vi "Click Cycle_Update Value.vi"(7 "Action":T1, 8 "Error In":errorcluster, 9 "Save Action":T2(ring)=enum."Remove", 10 "Tag":string, 11 "Row RW State":T3) -> (0 "Error Out":errorcluster)   [LabVIEW 2023]
uses:
  controls/action enum.ctl
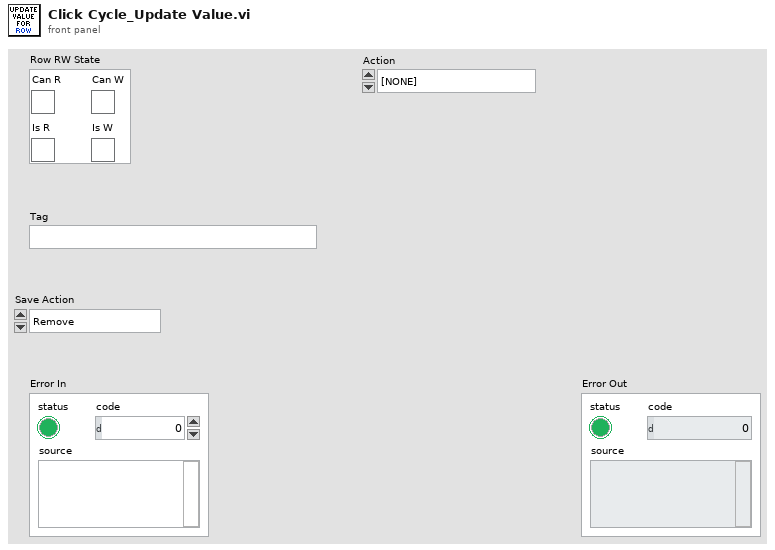
[diagram p1: front panel]
types:
  T1 = typedef "action enum.ctl" = enum16{"[NONE]", "Wire Bundle", "Wire Unbundle", "Terminal Unbundle", "Terminal Bundle", "Bundler Move Up", "Bundler Move Down", "Bundler Insert", "Bundler Remove", "Bundler Remove Unwired", "Bundler Rearrange", "In Place Insert", "In Place Remove", "In Place Remove Unwired", "In Place Rearrange", "Wire Properties", "Wire Method", "Terminal Properties", "Terminal Method", "Property Move Up", "Property Move Down", "Properties Insert", "Properties Remove", "Properties Remove Unwired", "Properties Rearrange", "Method Change", "Class for Constant", "Class For Control", "Class For Node", "Class Name to Clipboard"}
  T2 = enum16{"Init", "Read", "Remove", "Remove or Append", "Append", "Append If New"}
  T3 = cluster{"Can R":bool, "Can W":bool, "Is R":bool, "Is W":bool}
  T4 = cluster{"Tag":string, "Read":bool, "Write":bool, "New":bool}
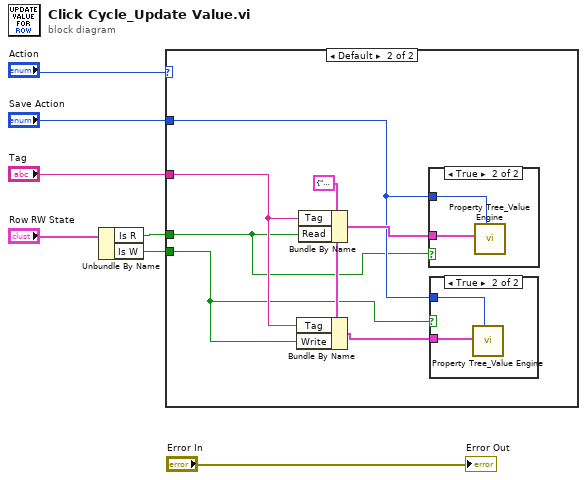
[diagram p0: block diagram]
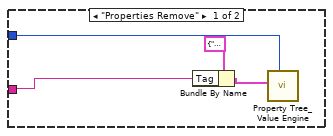
[diagram p2: hidden frame]
diagram:
  n1 = Unbundle By Name("Row RW State") -> ("Is R"=w4:bool, "Is W"=w3:bool)
  n2 = case shown="Default" "Action" {
    tunnel: "Tag" -> [w9 w16]
    tunnel: "Save Action" -> [w11 w14]
    tunnel: w4 -> [_ w13]
    tunnel: w3 -> [_ w12]
    frame "Properties Remove" {
      n3 = Bundle By Name(cluster=T4 {"Tag"="", "Read"=FALSE, "Write"=FALSE, "New"=FALSE} ("Element"), "Tag"=w9) -> (w8:T4)
      n4 = call "Property Tree_Value Engine.vi"("Save Action"=w11, "Element"=w8) -> ()  [unwired: 7 in, 3 out]
    }
    frame Default {
      w17 = T4 {"Tag"="", "Read"=FALSE, "Write"=FALSE, "New"=FALSE} ("Element")
      n5 = Bundle By Name(cluster=w17, "Tag"=w16, "Write"=w12) -> (w15:T4)
      n6 = Bundle By Name(cluster=w17, "Tag"=w16, "Read"=w13) -> (w18:T4)
      n7 = case shown="True" w13 {
        tunnel: w18 -> [_ w22]
        tunnel: w14 -> [_ w21]
        frame False {
        }
        frame True {
          n8 = call "Property Tree_Value Engine.vi"("Save Action"=w21, "Element"=w22) -> ()  [unwired: 7 in, 3 out]
        }
      }
      n9 = case shown="True" w12 {
        tunnel: w15 -> [_ w20]
        tunnel: w14 -> [_ w19]
        frame False {
        }
        frame True {
          n10 = call "Property Tree_Value Engine.vi"("Save Action"=w19, "Element"=w20) -> ()  [unwired: 7 in, 3 out]
        }
      }
    }
  }
  "Error Out" <- "Error In"
